vi "DisplayExecution Event Callback.vi"(4 "GUI.lvlib:Auto UI.lvlib:Auto UI.lvclass":refnum<class "Auto UI.lvclass">, 5 "Event data":cluster{"exec":refnum<k7>, "reason":i32}, 6 "CtlRef":refnum<k7>, 7 "Event common data":cluster{"Source":i32, "Type":u32, "Time":u32}) -> ()   [LabVIEW 2023, in "GUI.lvlib" / "Auto UI.lvlib" / "Auto UI.lvclass"]
uses:
  Auto UI.lvclass
  Auto UI.lvclass/Auto UI.ctl
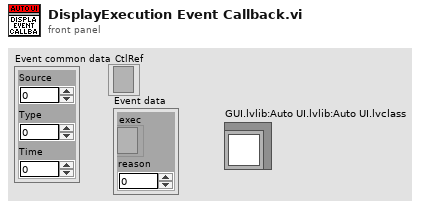
[diagram p1: front panel]
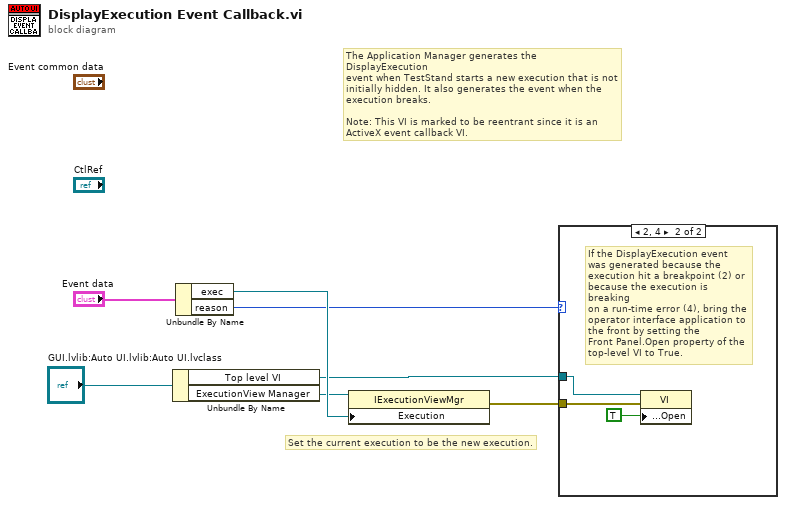
[diagram p0: block diagram]
diagram:
  # "The Application Manager generates the DisplayExecution\nevent when TestStand starts a new execution that is not\ninitially hidden. It also generates the event when the\nexecution breaks.\n\nNote: This VI is marked to be reentrant since it is an\nActiveX event callback VI."
  # "Set the current execution to be the new execution."
  n1 = Unbundle By Name("GUI.lvlib:Auto UI.lvlib:Auto UI.lvclass") -> ("Top level VI"=w3:refnum<vi>, "ExecutionView Manager"=w4:refnum<k7>)
  n2 = Unbundle By Name("Event data") -> ("exec"=w7:refnum<k7>, "reason"=w5:i32)
  n3 = property class="IExecutionViewMgr"(reference=w4, "Execution"=w7) -> (error out=w2:errorcluster)  [unwired: 1 in, 1 out]
  n4 = case shown="2, 4" w5 {
    tunnel: w2 -> [_ w10]
    tunnel: w3 -> [_ w8]
    frame Default {
    }
    frame 2, 4 {
      # "If the DisplayExecution event\nwas generated because the\nexecution hit a breakpoint (2) or\nbecause the execution is breaking\non a run-time error (4), bring the\noperator interface application to\nthe front by setting the\nFront Panel.Open property of the\ntop-level VI to True."
      n5 = property class="VI"(reference=w8, error in=w10, "Front Panel Window:Open"=TRUE) -> ()  [unwired: 2 out]
    }
  }
